vi "CreateSignalArray.vi"(4 "error in (no error)":errorcluster, 6 "bufferSize":dbl) -> (0 "error out":errorcluster)   [LabVIEW 2016]
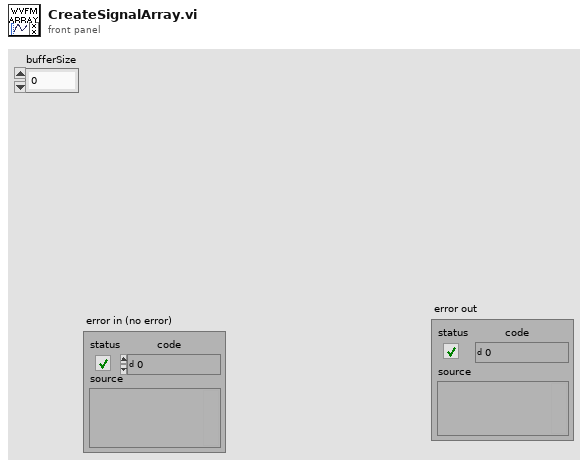
[diagram p1: front panel]
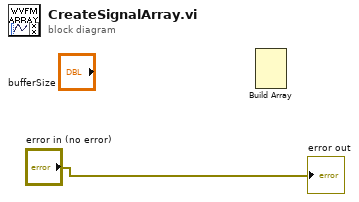
[diagram p0: block diagram]
diagram:
  n1 = Build Array() -> ()  [unwired: 5 in, 1 out]
  "error out" <- "error in (no error)"
